vi "Write Owner ID.vi"(8 "error in (no error)":errorcluster, 10 "Owner ID":string, 11 "Data Item in":refnum<class "Data Item.lvclass">) -> (0 "error out":errorcluster, 3 "Data Item out":refnum<class "Data Item.lvclass">)   [LabVIEW 2026, in "VILab.lvlib" / "Data Item.lvclass"]
uses:
  Data Item.lvclass
  Data Item.lvclass/Data Item.ctl
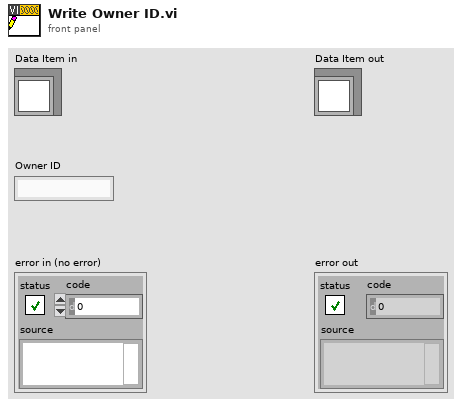
[diagram p1: front panel]
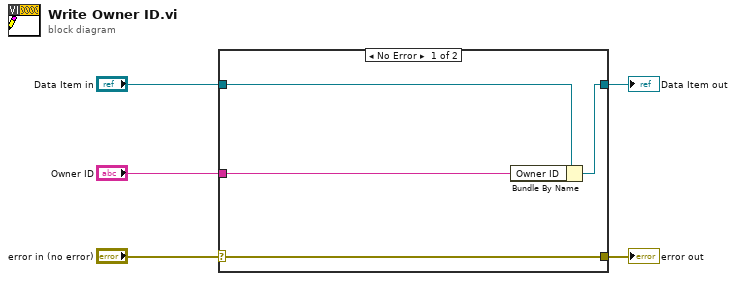
[diagram p0: block diagram]
diagram:
  n1 = case shown="No Error" "error in (no error)" {
    selector: "error in (no error)" -> [w9 w10]
    tunnel: [w9 w10] -> w4
    tunnel: [w7 w11] -> w2
    tunnel: "Data Item in" -> [w8 w11]
    tunnel: "Owner ID" -> [w6 _]
    frame No Error {
      n2 = Bundle By Name(cluster=w8, "Owner ID"=w6) -> (w7:refnum<class "Data Item.lvclass">)
    }
    frame Error {
    }
  }
  "error out" <- w4
  "Data Item out" <- w2
